vi "float-string converter.vi"(3 "float string in":string[](array[string]), 5 "float in":dbl[](array[numeric])) -> (0 "float out":dbl[](array[numeric]), 2 "float string out":string[](array[string]))   [LabVIEW 2015]
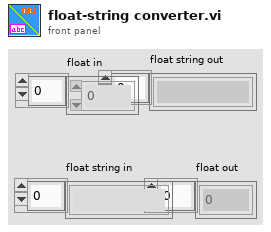
[diagram p1: front panel]
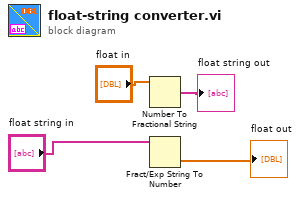
[diagram p0: block diagram]
diagram:
  n1 = Number To Fractional String(number="float in") -> (F-format string=→"float string out":string[])  [unwired: 3 in]
  n2 = Fract/Exp String To Number(string="float string in") -> (number=→"float out":dbl[])  [unwired: 3 in, 1 out]
